vi "Calculate Retroparticle Scores.vi"(9 "Aspect Fudge Factor":dbl=1.0, 10 "Sorted Data":dbl[][](array[numeric]), 11 "Image in":T2) -> (3 "Scores":T1(array[cluster]))   [LabVIEW 2014]
doc: "Calculate scores based on the particle measurements. Example scores are for trapezoidal area, aspect ratio, ratio of area to convex hull area, and masking for _| |_ shapes. These scores can later help to categorize particles into nonTargets, long targets, and short targets. The fudge factor compensates for camera modes that do not give square pixels."
uses:
  <vilib>/vision/Image Controls.llb/IMAQ Image.ctl
  <vilib>/vision/NI_Vision_Development_Module.lvlib
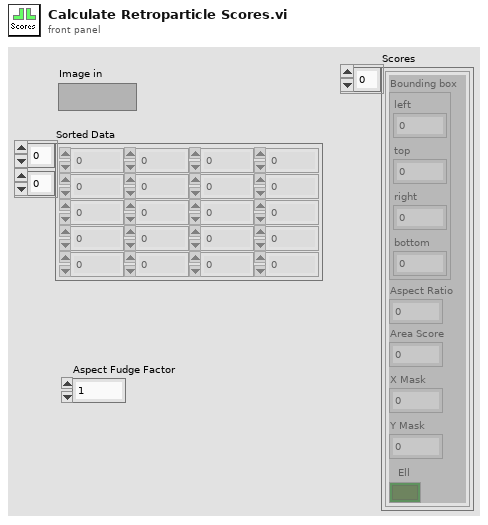
[diagram p1: front panel]
types:
  T1 = cluster{"Bounding box":cluster{"left":dbl, "top":dbl, "right":dbl, "bottom":dbl}, "Aspect Ratio":dbl, "Area Score":dbl, "X Mask":dbl, "Y Mask":dbl, "Ell":bool}[]
  T2 = typedef "IMAQ Image.ctl" = refnum<image>
  T3 = cluster{"[0]":dbl, "[1]":dbl, "[2]":dbl, "[3]":dbl}
  T4 = cluster{cluster{"[0]":dbl, "[1]":dbl, "[2]":dbl, "[3]":dbl}, "Score":dbl, "Score":dbl, "X Score":dbl, "Y Score":dbl, "Ell":bool}
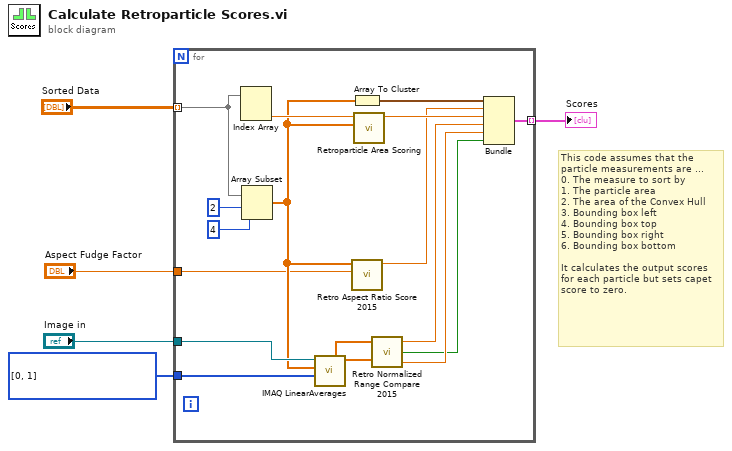
[diagram p0: block diagram]
diagram:
  w3 = i32[] [0, 1] items=["X Axis Averages", "Y Axis Averages", "X + Y Axis Averages", "X - Y Axis Averages"] ("Averages")
  # "This code assumes that the\nparticle measurements are ...\n0. The measure to sort by\n1. The particle area\n2. The area of the Convex Hull\n3. Bounding box left\n4. Bounding box top\n5. Bounding box right\n6. Bounding box bottom\n\nIt calculates the output scores\nfor each particle but sets capet\nscore to zero."
  n1 = for {
    tunnel: "Image in" -> [w18]
    tunnel: "Sorted Data" -> [w20] mode=indexing
    tunnel: [w19] -> w4 mode=indexing
    tunnel: w3 -> [w16]
    tunnel: "Aspect Fudge Factor" -> [w12]
    n2 = Index Array(array=w20) -> (element #2=w15:dbl)  [unwired: 2 in, 1 out]
    n3 = Array Subset(array=w20, index=2, length=4) -> (w13:dbl[])
    n4 = call "IMAQ LinearAverages"("Averages"=w16, "Optional Rectangle"=w13, "Image Src"=w18) -> ("Y Axis Averages"=w7:sgl[], "X Axis Averages"=w8:sgl[])  [unwired: 4 in, 3 out]
    n5 = Array To Cluster(array=w13) -> (cluster=w17:T3)
    n6 = call "Retro Aspect Ratio Score 2015.vi"("Aspect Fudge Factor"=w12, "Rectangle Array ltrb"=w13) -> ("Score"=w11:dbl)  [unwired: 9 in]
    n7 = call "Retroparticle Area Scoring.vi"("Rectangle Array ltrb"=w13, "Particle Area"=w15) -> ("Score"=w14:dbl)  [unwired: 9 in]
    n8 = call "Retro Normalized Range Compare 2015.vi"("Y Averages"=w7, "X Averages"=w8) -> ("Y Score"=w9:dbl, "Ell"=w6:bool, "X Score"=w10:dbl)  [unwired: 1 in]
    n9 = Bundle(w17, "Score"=w11, "Score"=w14, "X Score"=w10, "Y Score"=w9, "Ell"=w6) -> (w19:T4)  [unwired: 1 in]
  }
  "Scores" <- w4
